vi "Write Handle Drag Over Msg.vi"(6 "Handle Drag Over Msg":refnum<class "Handle Drag Over Msg.lvclass">, 11 "Test Executive Builder Event Filter in":refnum<class "Test Executive Builder Event Filter.lvclass">) -> (3 "Test Executive Builder Event Filter out":refnum<class "Test Executive Builder Event Filter.lvclass">)   [LabVIEW 2017, in "Test Executive Builder Event Filter.lvclass"]
uses:
  <vilib>/gpm_packages/@cs/Test-executive-builder/Source/Test Executive Builder View/Test Executive Builer Event Filter/Test Executive Builder Event Filter.lvclass
  <vilib>/gpm_packages/@cs/Test-executive-builder/Source/Test Executive Builder View/Test Executive Builder View Messages/Handle Drag Over Msg/Handle Drag Over Msg.lvclass
  <vilib>/gpm_packages/@cs/Test-executive-builder/Source/Test Executive Builder View/Test Executive Builer Event Filter/Test Executive Builder Event Filter.lvclass/Test Executive Builder Event Filter.ctl
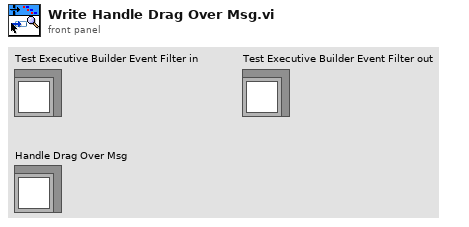
[diagram p1: front panel]
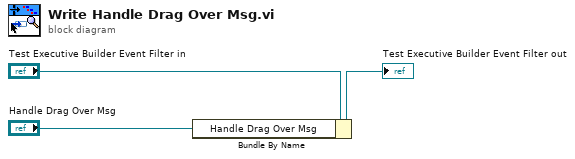
[diagram p0: block diagram]
diagram:
  n1 = Bundle By Name(cluster="Test Executive Builder Event Filter in", "Handle Drag Over Msg"="Handle Drag Over Msg") -> (→"Test Executive Builder Event Filter out":refnum<class "Test Executive Builder Event Filter.lvclass">)
